vi "High Sampling waste.vi"() -> ()   [LabVIEW 2025]
panel:
  out "Plot Title 5":dbl[](graph)
  out "Plot Title 4":dbl[](graph)
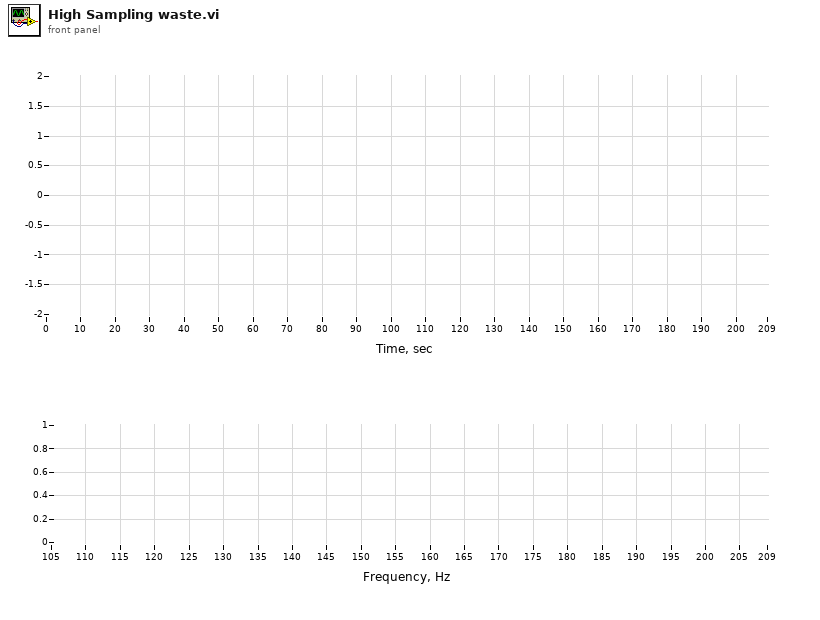
[diagram p1: front panel]
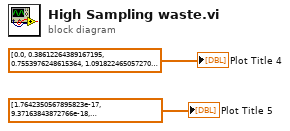
[diagram p0: block diagram]
diagram:
  "Plot Title 4" <- dbl[] [0.0, 0.38612264389167195, 0.7553976248615364, 1.0918224650572705, 1.3810394437280533, 1.6110464864151235, 1.7727812442359645, 1.8605472991527119, 1.8722602153051073, 1.8095011659031264, 1.6773765349520993, 1.4841926215855477, 1.2409647577484988, 0.960789214813603, 0.6581137129666796, 0.34794774335047207, 0.04505696792874103, -0.23681348994758378, -0.4856440334338919, -0.6917354195126166, -0.8481615310050049, -0.9510565162951529, -0.9997223318635131, -0.996553077294895, -0.9467830165234634, -0.8580752324745258, -0.7399768917159529, -0.6032745876693928, -0.4592887607086381, -0.3191494495291979, -0.19309642971379382, -0.08984510261331546, -0.01605541378700792, 0.024065154359490748, 0.029001492898684034, -4.440892098500626e-16, -0.05903661864063936, -0.14182212168023767, -0.24011040060916328, -0.34424443021412543, -0.44379744058708, -0.5282677288291038, -0.5877852522924745, -0.6137873056860932, -0.5996222332554337, -0.5410441730642667, -0.43656804374665226, -0.2876620106797483, -0.09876404938870875, 0.12288057830704324, 0.36755369058058196, 0.62355308810048, 0.8778095726409358, 1.116598021721424, 1.3263027362631667, 1.4941938067078262, 1.6091702292618337, 1.6624270143247684, 1.6480074862215872, 1.5632081598738967, 1.4088116512993833, 1.1891325820772427, 0.911871838038443, 0.5877852522924752, 0.23018319647675606, -0.1457129082347275, -0.5235230480209896, -0.8865297155180798, -1.2185233538616, -1.5046263462954195, -1.7320508075688763, -1.890748990187092, -1.9739209787231378, -1.9783521805753521, -1.9045624917490453, -1.7567593946498536, -1.5425980477592118, -1.2727620468602399, -0.9603883772666684, -0.620368583825887, -0.2685648836527202, 0.07901553828834562, 0.4070427284730844, 0.7016377995111623, 0.9510565162951508, 1.1462460633573517, 1.281245768334423, 1.3534115116690062, 1.3634536060748261, 1.315288507613096, 1.2157152215855864, 1.0739370946021967, 0.900958282474805, 0.7088910666151479, 0.510214972776813, 0.317031059410261, 0.14035465846052197, -0.010512718016697842, -0.12849649158383292, -0.20911827929990312, -0.25070101087328256, -0.25439932760080697, -0.22405498682215186, -0.16588727603972547, -0.08803811153932023, 2.7200464103316335e-15, 0.08803811153932589, 0.16588727603973075, 0.22405498682215713, 0.25439932760081185, 0.2507010108732871, 0.20911827929990712, 0.12849649158383636, 0.010512718016700506, -0.14035465846051998, -0.3170310594102599, -0.5102149727768128, -0.7088910666151484, -0.9009582824748067, -1.0739370946021989, -1.2157152215855898, -1.3152885076131, -1.363453606074831, -1.3534115116690115, -1.2812457683344292, -1.1462460633573581, -0.9510565162951574, -0.7016377995111691, -0.4070427284730911, -0.07901553828835223, 0.2685648836527142, 0.6203685838258813, 0.9603883772666635, 1.2727620468602356, 1.542598047759209, 1.7567593946498514, 1.9045624917490445, 1.9783521805753521, 1.973920978723139, 1.8907489901870944, 1.7320508075688794, 1.504626346295424, 1.2185233538616052, 0.8865297155180859, 0.5235230480209958, 0.14571290823473448, -0.23018319647674929, -0.587785252292468, -0.9118718380384363, -1.189132582077236, -1.4088116512993776, -1.563208159873891, -1.6480074862215823, -1.6624270143247646, -1.6091702292618306, -1.4941938067078246, -1.3263027362631654, -1.1165980217214244, -0.8778095726409363, -0.6235530881004823, -0.3675536905805842, -0.12288057830704713, 0.09876404938870498, 0.2876620106797433, 0.43656804374664715, 0.541044173064261, 0.5996222332554277, 0.6137873056860872, 0.5877852522924681, 0.5282677288290982, 0.4437974405870739, 0.3442444302141204, 0.2401104006091579, 0.14182212168023356, 0.05903661864063503, -2.4424906541753444e-15, -0.02900149289868681, -0.024065154359492302, 0.016055413787006922, 0.08984510261331535, 0.1930964297137947, 0.3191494495291992, 0.45928876070864083, 0.6032745876693957, 0.7399768917159573, 0.85807523247453, 0.9467830165234691, 0.9965530772949002, 0.9997223318635196, 0.9510565162951587, 0.8481615310050115, 0.6917354195126226, 0.485644033433898, 0.23681348994758933, -0.045056967928735925, -0.3479477433504674, -0.6581137129666759, -0.9607892148135997, -1.2409647577484968, -1.4841926215855459, -1.6773765349520997, -1.8095011659031266, -1.8722602153051096, -1.860547299152714, -1.7727812442359685, -1.6110464864151277, -1.3810394437280586, -1.091822465057276, -0.755397624861543, -0.3861226438916783] ("The Signal")
  "Plot Title 5" <- dbl[] [1.7642350567895823e-17, 9.37163843872766e-18, 8.957717334525772e-18, 6.130247306098902e-17, 3.115986551573719e-17, 9.991544958444242e-17, 3.8667772806554363e-17, 2.3386367327236014e-17, 1.0697783918221356e-16, 4.9331385463801225e-17, 7.404553746064768e-17, 1.8542802640634544e-17, 1.768133757748647e-17, 1.5516195773292916e-17, 1.0274204839244388e-17, 1.3381613584971875e-17, 3.459006278307491e-18, 2.0753141198503237e-17, 1.2455756516521877e-17, 1.666631907138501e-17, 5.3803433635825707e-17, 1.3755652082361817e-17, 2.4627141816828866e-17, 5.2971372556679015e-17, 1.4256740398966348e-17, 2.100758603565018e-17, 3.391533731641999e-17, 1.0958974031744888e-17, 2.3562312665717715e-17, 1.959808683334833e-17, 3.998462922807662e-17, 1.1830740209957694e-17, 2.858937966027981e-17, 2.327245184639182e-17, 2.3697212394211837e-17, 1.4908802924697426e-17, 6.811148557205684e-18, 3.531097827590309e-17, 8.6119184938481e-18, 1.651253138484665e-17, 7.82449883721225e-17, 3.458704393110099e-17, 1.0373771372973356e-17, 5.0982843490520985e-17, 2.9510197115073305e-17, 2.4033497896183676e-17, 2.8316757861758615e-17, 9.773868470677327e-17, 1.8961351982703756e-17, 2.9695399960343195e-17, 1.4185168446233834e-16, 1.8538800144157063e-17, 2.6301603220229034e-17, 2.5637942661149868e-17, 2.390871264020655e-17, 3.324349123645815e-17, 1.8603732275468945e-17, 4.788579196861479e-17, 3.6155014039054835e-17, 2.066061264806352e-17, 5.746679005008987e-17, 3.356619189690116e-17, 3.1521851245023783e-17, 2.631023821598099e-17, 3.534249192672814e-17, 1.5641767257388586e-17, 4.161587175097087e-17, 4.9726605133469926e-17, 2.985203037225326e-17, 3.332939525513794e-17, 1.2525790172773125e-17, 3.939813782169714e-17, 4.287619099498766e-17, 6.757316332078684e-17, 4.300276403402975e-17, 4.430337328543282e-17, 4.073737057547146e-17, 5.991375871476371e-17, 4.621425971516324e-17, 3.5664155370786714e-17, 1.3534281137232882e-16, 3.9376632592972707e-17, 3.882076355120276e-17, 4.8776304368288834e-17, 5.60864371135822e-17, 6.141984110076596e-17, 6.166516026876021e-17, 8.768405916261646e-17, 6.83693148506251e-17, 8.563679705444875e-17, 3.168046113777112e-16, 9.846719285674402e-17, 8.710245204618101e-17, 1.8792555601230047e-16, 1.4658959607432608e-16, 1.436871336182269e-16, 2.1256278699589125e-16, 0.5, 2.654144290910317e-16, 5.647152065653281e-16, 0.5, 4.501885091602085e-16, 2.0466850674991302e-16, 1.2340293269478133e-16, 6.111751206251929e-17, 1.559599010782958e-17, 6.111751206251929e-17, 1.2340293269478133e-16, 2.0466850674991302e-16, 4.501885091602085e-16, 0.5, 5.647152065653281e-16, 2.654144290910317e-16, 0.5, 2.1256278699589125e-16, 1.436871336182269e-16, 1.4658959607432608e-16, 1.8792555601230047e-16, 8.710245204618101e-17, 9.846719285674402e-17, 3.168046113777112e-16, 8.563679705444875e-17, 6.83693148506251e-17, 8.768405916261646e-17, 6.166516026876021e-17, 6.141984110076596e-17, 5.60864371135822e-17, 4.8776304368288834e-17, 3.882076355120276e-17, 3.9376632592972707e-17, 1.3534281137232882e-16, 3.5664155370786714e-17, 4.621425971516324e-17, 5.991375871476371e-17, 4.073737057547146e-17, 4.430337328543282e-17, 4.300276403402975e-17, 6.757316332078684e-17, 4.287619099498766e-17, 3.939813782169714e-17, 1.2525790172773125e-17, 3.332939525513794e-17, 2.985203037225326e-17, 4.9726605133469926e-17, 4.161587175097087e-17, 1.5641767257388586e-17, 3.534249192672814e-17, 2.631023821598099e-17, 3.1521851245023783e-17, 3.356619189690116e-17, 5.746679005008987e-17, 2.066061264806352e-17, 3.6155014039054835e-17, 4.788579196861479e-17, 1.8603732275468945e-17, 3.324349123645815e-17, 2.390871264020655e-17, 2.5637942661149868e-17, 2.6301603220229034e-17, 1.8538800144157063e-17, 1.4185168446233834e-16, 2.9695399960343195e-17, 1.8961351982703756e-17, 9.773868470677327e-17, 2.8316757861758615e-17, 2.4033497896183676e-17, 2.9510197115073305e-17, 5.0982843490520985e-17, 1.0373771372973356e-17, 3.458704393110099e-17, 7.82449883721225e-17, 1.651253138484665e-17, 8.6119184938481e-18, 3.531097827590309e-17, 6.811148557205684e-18, 1.4908802924697426e-17, 2.3697212394211837e-17, 2.327245184639182e-17, 2.858937966027981e-17, 1.1830740209957694e-17, 3.998462922807662e-17, 1.959808683334833e-17, 2.3562312665717715e-17, 1.0958974031744888e-17, 3.391533731641999e-17, 2.100758603565018e-17, 1.4256740398966348e-17, 5.2971372556679015e-17, 2.4627141816828866e-17, 1.3755652082361817e-17, 5.3803433635825707e-17, 1.666631907138501e-17, 1.2455756516521877e-17, 2.0753141198503237e-17, 3.459006278307491e-18, 1.3381613584971875e-17, 1.0274204839244388e-17, 1.5516195773292916e-17, 1.768133757748647e-17, 1.8542802640634544e-17, 7.404553746064768e-17, 4.9331385463801225e-17, 1.0697783918221356e-16, 2.3386367327236014e-17, 3.8667772806554363e-17, 9.991544958444242e-17, 3.115986551573719e-17, 6.130247306098902e-17, 8.957717334525772e-18, 9.37163843872766e-18] ("The Spectrum")
